vi "Flip Flop JK (2).vi"() -> ()   [LabVIEW 2018]
panel:
  out "Q2*":bool
  in  "Q2":bool
  in  "K":bool
  in  "J":bool
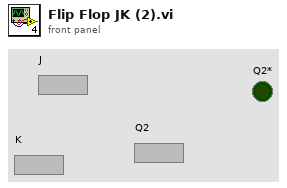
[diagram p1: front panel]
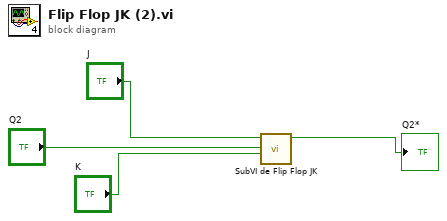
[diagram p0: block diagram]
diagram:
  n1 = call "SubVI de Flip Flop JK.vi"("K"="K", "Q2"="Q2", "J"="J") -> ("Q2*"=→"Q2*":bool)  [unwired: 8 in]
